vi "RN_Motor_Schrittgeschwindigkeit.vi"(6 "error in":errorcluster, 7 "Schrittgeschwindigkeit":u8=9, 8 "Motorwahl":string(combo)="0", 9 "VISA resource name in":refnum<visa-resource-name>) -> (0 "error out":errorcluster, 2 "Gesendeter Code":string, 3 "VISA resource name out":refnum<visa-resource-name>)   [LabVIEW 2014]
doc: "VI zum Einstellen der Schrittgeschwindigkeit der Motoren der RN-Motorsteuerung;\n\nDie Schrittgeschwindigkeit wird in Stufen von 0 bis 255 eingestellt. 0 ist dabei die schnellste und 255 die langsamste Schjrittgeschwindigkeit. \n\n0= 1000 Schritte pro Sek.\n1= 500 Schritte pro Sek.\n2= 333 Schritte pro Sek.\n3= 250 Schritte pro Sek.\n4= 200 Schritte pro Sek.\n5= 167 Schritte pro Sek\n6= 142 Schritte pro Sek\n7= 125 Schritte pro Sek\n8= 111 Schritte pro Sek\n9= 100 Schritte pro Sek [Standard]\n...\n255= 4 Schritte pro Sekunde\n(geringe Abweichungen sind möglich)\n\nWichtig: Anzumerken ist noch, das nicht alle Schittmotoren die hohen Geschwindigkeitsstufen 0 bis 4 erlauben. Wenn sich der Motor bei diesen Stufen nicht dreht, so ist zu prüfen ob auch der zulässige Maximalstrom eingestellt ist. Ist dies der Fall und der Motor dreht immer noch nicht, dann ist die Geschwindigkeit zu hoch für den Motor."
panel:
  in  "Steuercode":string="g"
  in  "Kennung - RN-Motorsteuerung":string="#rm"
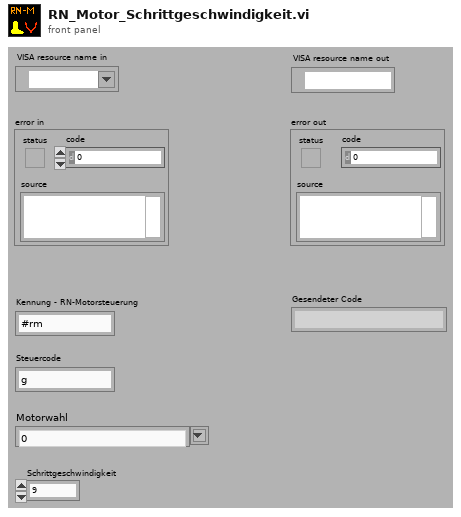
[diagram p1: front panel]
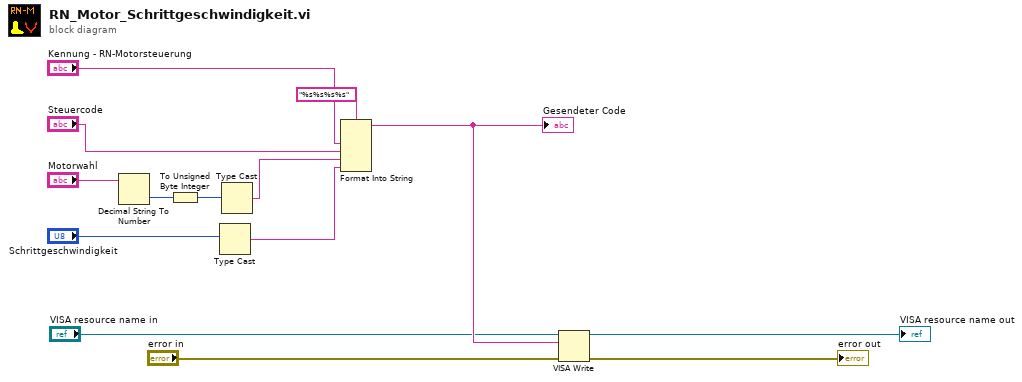
[diagram p0: block diagram]
diagram:
  n1 = Decimal String To Number(string="Motorwahl") -> (number=w13:i32)  [unwired: 2 in, 1 out]
  n2 = To Unsigned Byte Integer(number=w13) -> (unsigned 8bit integer=w12:u8)
  n3 = Type Cast(x="Schrittgeschwindigkeit") -> (*(type *) &x=w7:string)  [unwired: 1 in]
  n4 = Type Cast(x=w12) -> (*(type *) &x=w8:string)  [unwired: 1 in]
  n5 = Format Into String(format string="%s%s%s%s", "Kennung - RN-Motorsteuerung", "Steuercode", w8, w7) -> (resulting string=w5:string)  [unwired: 2 in, 1 out]
  "Gesendeter Code" <- w5
  n6 = VISA Write(VISA resource name="VISA resource name in", write buffer=w5, error in (no error)="error in") -> (VISA resource name out=→"VISA resource name out":refnum<visa-resource-name>, error out=→"error out":errorcluster)  [unwired: 1 out]
